vi "Stepper Pulse Generator.vi"(11 "Tick Count":i32) -> ()   [LabVIEW 2018]
uses:
  <vilib>/Platform/TimedLoop/XDataNode/timing_clust.ctl
  <vilib>/Platform/TimedLoop/XDataNode/nitl_modes.ctl
  <vilib>/Platform/TimedLoop/XDataNode/wakeup.ctl
  <vilib>/rvi/Emulation/niFpgaSctlEmulationGetInTimedLoop.vi
  <vilib>/rvi/Emulation/niFpgaEmulationReportErrorSimple.vi
  <vilib>/rvi/Emulation/niFpgaGetClockAttributes.vi
  <vilib>/rvi/Emulation/niFpgaCriticalErrorInLSC.vi
  <vilib>/rvi/eio/common/nirviEmuTemplateMethod_errors.vi
  <vilib>/rvi/Emulation/niFpgaProcessEmulError.vi
  <vilib>/Platform/TimedLoop/XDataNode/XDataNode.xnode
  <vilib>/eio/EIONode/EIONode.xnode
  <vilib>/Platform/TimedLoop/XDataNode/XDNodeRunTimeDep.lvlib
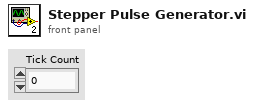
[diagram p1: front panel]
types:
  T1 = typedef "XDNodeRunTimeDep.lvlib/timing_clust.ctl" = cluster{"Expected End [f-1]":u64, "Actual End [f-1]":u64, "Finished Late? [f-1]":bool, "Expected End [i-1]":u64, "Actual End [i-1]":u64, "Finished Late? [i-1]":bool, "Expected Start [i]":u64, "Actual Start [i]":u64, "Expected Start [f]":u64, "Actual Start [f]":u64, "Source Name":string, "Structure Name":string, "Period":i64, "Deadline":i64, "Offset":i64, "Start":i64, "Priority":i32, "Timeout":i32, "Mode":T2, "Wakeup Reason":T3, "Error":errorcluster, "Source Type":string, "Secondary Source Type":string, "Global End Time":u64, "Global Start Time":u64, "Frame Duration":u64, "Iteration Duration":u64, "Assigned CPU":i32, "I/O Scan Engine Mode":u32}
  T2 = typedef "XDNodeRunTimeDep.lvlib/nitl_modes.ctl" = enum32{"No Change", "Process missed periods, maintain original phase", "Discard missed periods, maintain original phase", "Process missed periods, ignore original phase", "Discard missed periods, ignore original phase"}
  T3 = typedef "XDNodeRunTimeDep.lvlib/wakeup.ctl" = enum32{"Normal", "Aborted", "Asynchronous wakeup", "Timing source error", "Timed loop error", "Timeout"}
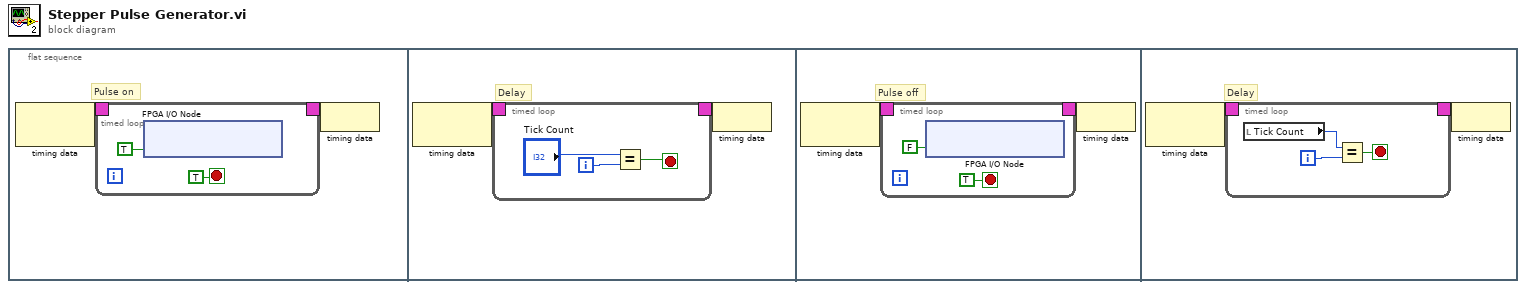
[diagram p0: block diagram]
diagram:
  n1 = flat-sequence {
    frame #0 {
      # "Pulse on"
      n2 = node-c288() -> (w2:T1)  [unwired: 1 in]
      n3 = timed-loop {
        timing: w2 -> [_]
        timing-out: [_] -> w1
        stop <- TRUE stop-if-true
        n4 = xnode "FPGA I/O Node"("ConnectorA/DIO0"=TRUE ("Connector0/DIO0")) -> ()  [unwired: 1 in, 1 out]
      }
      n5 = node-c288(w1) -> ()
    }
    frame #1 {
      # "Delay"
      n6 = node-c288() -> (w10:T1)  [unwired: 1 in]
      n7 = timed-loop {
        timing: w10 -> [_]
        timing-out: [_] -> w9
        i -> [w13]
        stop <- w11 stop-if-true
        n8 = Equal?(x="Tick Count", y=w13) -> (x = y?=w11:bool)
      }
      n9 = node-c288(w9) -> ()
    }
    frame #2 {
      # "Pulse off"
      n10 = node-c288() -> (w19:T1)  [unwired: 1 in]
      n11 = timed-loop {
        timing: w19 -> [_]
        timing-out: [_] -> w18
        stop <- TRUE stop-if-true
        n12 = xnode "FPGA I/O Node"("ConnectorA/DIO0"=FALSE ("Connector0/DIO0")) -> ()  [unwired: 1 in, 1 out]
      }
      n13 = node-c288(w18) -> ()
    }
    frame #3 {
      # "Delay"
      n14 = node-c288() -> (w27:T1)  [unwired: 1 in]
      n15 = timed-loop {
        timing: w27 -> [_]
        timing-out: [_] -> w26
        i -> [w30]
        stop <- w28 stop-if-true
        n16 = local read "Tick Count"() -> (w29:i32)
        n17 = Equal?(x=w29, y=w30) -> (x = y?=w28:bool)
      }
      n18 = node-c288(w26) -> ()
    }
  }
